vi "ConvertGP275Bytes.vi"(1 "Device Input Cluster":T1={"Dnet"="", "Node"=0, "Type"="", "ID Number"=0, "SCCM"=0.0, "FullScale"=0.0, "Input Bytes"=0, "Output Bytes"=0, "Input Start Location"=0, "Output Start Location"=0, "Enabled"=TRUE, "Bytes"=[]}) -> (0 "Device Output Cluster":T1={"Dnet"="", "Node"=0, "Type"="", "ID Number"=0, "SCCM"=0.0, "FullScale"=0.0, "Input Bytes"=0, "Output Bytes"=0, "Input Start Location"=0, "Output Start Location"=0, "Enabled"=TRUE, "Bytes"=[]})   [LabVIEW 2011]
uses:
  Excel/Device Cluster.ctl
  GlobalVariables.vi
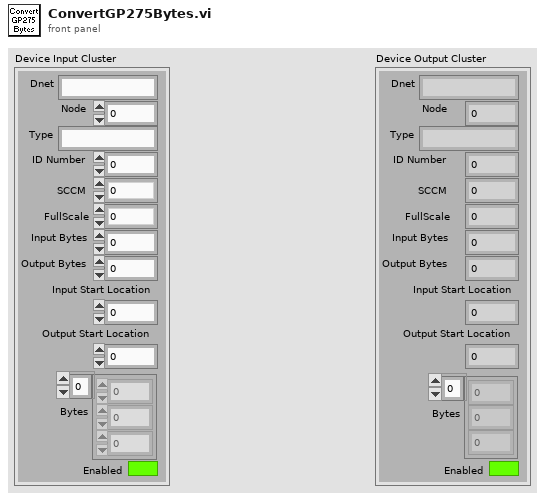
[diagram p1: front panel]
types:
  T1 = typedef "Device Cluster.ctl" = cluster{"Dnet":string, "Node":i32, "Type":string, "ID Number":u8, "SCCM":dbl, "FullScale":dbl, "Input Bytes":i32, "Output Bytes":i32, "Input Start Location":i32, "Output Start Location":i32, "Enabled":bool, "Bytes":u8[]}
  T2 = typedef "GP275 Cluster.ctl" = cluster{"Pressure (Torr)":sgl}
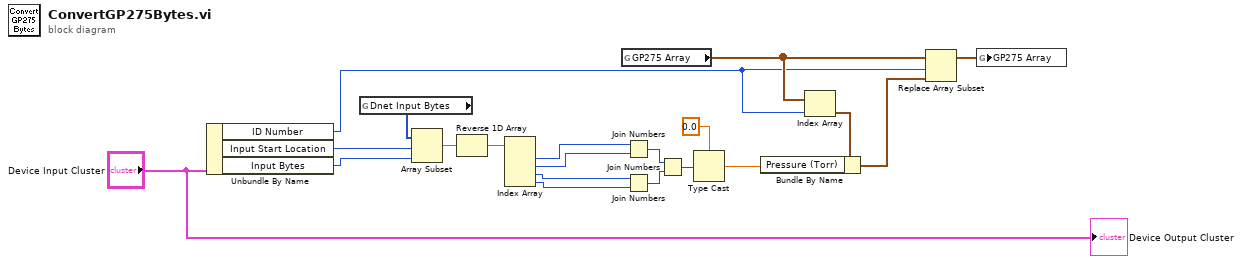
[diagram p0: block diagram]
diagram:
  n1 = Unbundle By Name("Device Input Cluster") -> ("ID Number"=w1:u8, "Input Start Location"=w2:i32, "Input Bytes"=w3:i32)
  n2 = global read "GlobalVariables.vi" "Dnet Input Bytes"() -> (w16:u8[])
  n3 = Array Subset(array=w16, index=w2, length=w3) -> (w7:u8[])
  n4 = Reverse 1D Array(array=w7) -> (reversed array=w8:u8[])
  n5 = Index Array(array=w8) -> (element #1=w12:u8, element #2=w11:u8, element #3=w10:u8, element #4=w9:u8)  [unwired: 4 in]
  n6 = global read "GlobalVariables.vi" "GP275 Array"() -> (w5:T2[])
  n7 = Join Numbers(hi=w12, lo=w11) -> ((hi.lo)=w18:u16)
  n8 = Join Numbers(hi=w10, lo=w9) -> ((hi.lo)=w19:u16)
  n9 = Join Numbers(hi=w18, lo=w19) -> ((hi.lo)=w17:u32)
  n10 = Type Cast(type=sgl 0.0, x=w17) -> (*(type *) &x=w6:sgl)
  n11 = Index Array(array=w5, index=w1) -> (element=w15:T2)
  n12 = Bundle By Name(cluster=w15, "Pressure (Torr)"=w6) -> (w14:T2)
  n13 = Replace Array Subset(array=w5, new element=w14, index=w1) -> (w4:T2[])
  n14 = global write "GlobalVariables.vi" "GP275 Array"(w4) -> ()
  "Device Output Cluster" <- "Device Input Cluster"
